vi "Teleop.vi"(10 "Match Info":T1={"Autonomous Elapsed Seconds"=0.0, "TeleOp Elapsed Seconds"=0.0, "Disabled Elapsed Seconds"=0.0, "Visited Autonomous"=FALSE, "Visited TeleOp"=FALSE, "Visited Disabled"=FALSE, "Autonomous Settings"={"Autonomous Style"=enum."Independent", "VI Refnum"=refnum}}, 11 "Call Context":T2) -> ()   [LabVIEW 2014]
doc: "This VI is called for each TeleOp packet received from the DS where the robot is not disabled. It is often used to read from the joysticks and update I/O or to update setpoints for timed control loops. It should complete and return within 20 milliseconds or it may miss DS packets."
uses:
  <vilib>/Rock Robotics/WPI/DriverStation/WPI_DriverStationDerivedRobotMode.ctl
  <vilib>/Rock Robotics/WPI/DriverStation/WPI_DriverStationMatch Info.ctl
  <vilib>/Rock Robotics/WPI/Joystick/WPI_JoystickGetSetRefNum.vi
  <vilib>/Rock Robotics/Network Tables/SD Write Boolean Array.vi
  <vilib>/Rock Robotics/Network Tables/SD Write Numeric Array.vi
panel:
  out "Right Motor":dbl(graph)
  out "Left Motor":dbl(graph)
  out "Left Sensor Velocity":dbl
  out "Right Sensor Velocity":dbl
  out "Waveform Chart":dbl(graph)
  in  "SET VALUE":dbl
  in  "TRUE - JOY\nFALSE - SET VALUE":bool
  out "X Value":dbl
  out "Y value":dbl
  out "Right Sensor Velocity In inches per second 2":dbl(graph)
  out "Left Sensor Velocity In inches per second":dbl(graph)
  out "Applied Throttle":dbl(graph)
  out "Motor Output":dbl
  # "Sensor Velocity is in ticks per 100ms"
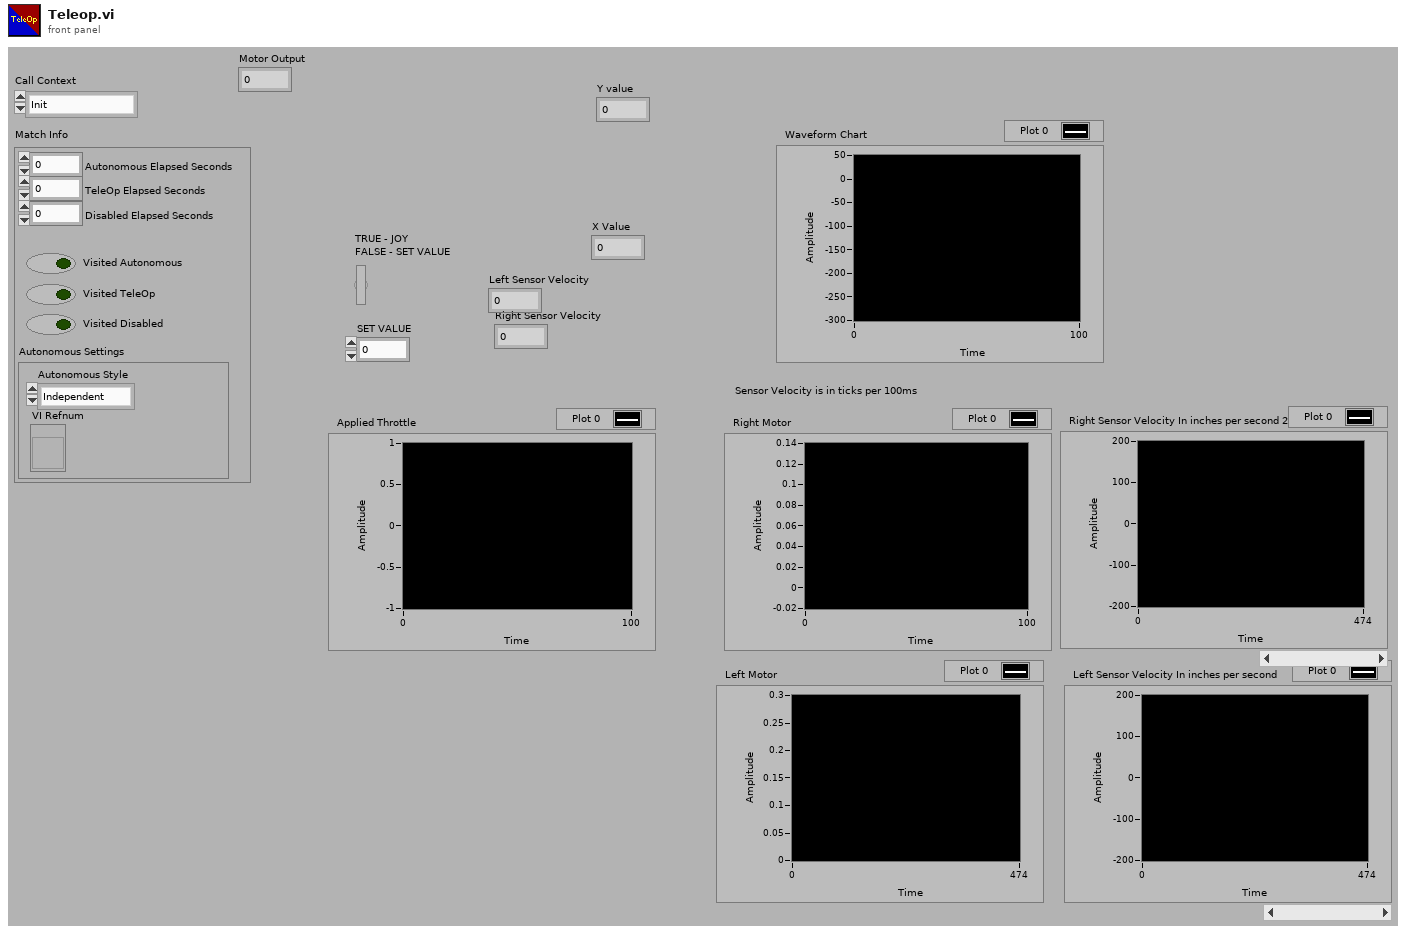
[diagram p1: front panel]
types:
  T1 = typedef "WPI_DriverStationMatch Info.ctl" = cluster{"Autonomous Elapsed Seconds":dbl, "TeleOp Elapsed Seconds":dbl, "Disabled Elapsed Seconds":dbl, "Visited Autonomous":bool, "Visited TeleOp":bool, "Visited Disabled":bool, "Autonomous Settings":cluster{"Autonomous Style":enum16{"Iterative", "Independent"}, "VI Refnum":refnum<vi>}}
  T2 = typedef "WPI_DriverStationDerivedRobotMode.ctl" = enum16{"Init", "Execute", "Stop"}
  T3 = typedef "WPI_MotorControlDeviceRef.ctl" = cluster{"DeviceStatus":errorcluster, "Type":T4, "PWM":cluster{"Controller":T5, "PWM Channel":T6, "DeadBand":T7}, "CAN":cluster{"Device Number":u8, "Control Mode":T8, "Semaphore":T9, "Max Vout":dbl, "TalonSRX Control Mode":T10}, "Invert":bool, "TransformRef":T11, "InvTransformRef":T11}
  T4 = typedef "WPI_MotorControlType.ctl" = enum16{"PWM", "CAN", "CANTalonSRX"}
  T5 = typedef "FPGA_TypedefDigitalModule.ctl" = enum16{"Controller 1"}
  T6 = typedef "FPGA_DIOPWMChannel.ctl" = enum8{"PWM 0", "PWM 1", "PWM 2", "PWM 3", "PWM 4", "PWM 5", "PWM 6", "PWM 7", "PWM 8", "PWM 9", "PWM MXP 0", "PWM MXP 1", "PWM MXP 2", "PWM MXP 3", "PWM MXP 4", "PWM MXP 5", "PWM MXP 6", "PWM MXP 7", "PWM MXP 8", "PWM MXP 9", "Invalid"}
  T7 = typedef "WPI_PWMDeadband.ctl" = cluster{"Name":string, "maxPositivePwm":i32, "minPositivePwm":i32, "centerPwm":i32, "maxNegativePwm":i32, "minNegativePwm":i32, "angularRange":u16}
  T8 = typedef "WPI_CANJaguar_ControlMode.ctl" = enum8{"Percent VBus", "Current", "Speed", "Position", "Voltage"}
  T9 = typedef "Semaphore RefNum" = refnum<k1>
  T10 = typedef "WPI_CANTalonSRX_APIControlMode.ctl" = enum8{"Percent VBus", "Speed", "Position", "Slave", "Unchanged / Invalid"}
  T11 = typedef "WPI_PWMTransform_ConPane.ctl" = refnum<vi>
  T12 = typedef "WPI_JoystickDevRef.ctl" = cluster{"Device":T13}
  T13 = typedef "WPI_JoystickDeviceEnum.ctl" = enum16{"USB 0", "USB 1", "USB 2", "USB 3", "USB 4", "USB 5"}
  T14 = typedef "WPI_CANTalonSRX_GlobalStatus.ctl" = cluster{"Applied Throttle":dbl, "Module Enabled":bool, "CAN Error":errorcluster, "Closed Loop Error":dbl, "Forward Limit Switch Closed":bool, "Reverse Limit Switch Closed":bool, "Sensor Position":dbl, "Sensor Velocity":dbl, "Current":dbl, "Sticky Fault - Over Temp":bool, "Sticky Fault - Under Voltage":bool, "Sticky Fault - Forward Limit":bool, "Sticky Fault - Reverse Limit":bool, "Sticky Fault - Forward Soft Limit":bool, "Sticky Fault - Reverse Soft Limit":bool, "Brake is Enabled":bool, "Encoder Position":dbl, "Encoder Velocity":dbl, "Encoder Index Count":dbl, "Encoder A Pin State":bool, "Encoder B Pin State":bool, "Encoder Index Pin State":bool, "Analog In":dbl, "Analog In Velocity":dbl, "Temperature (C)":dbl, "Battery Voltage":dbl}
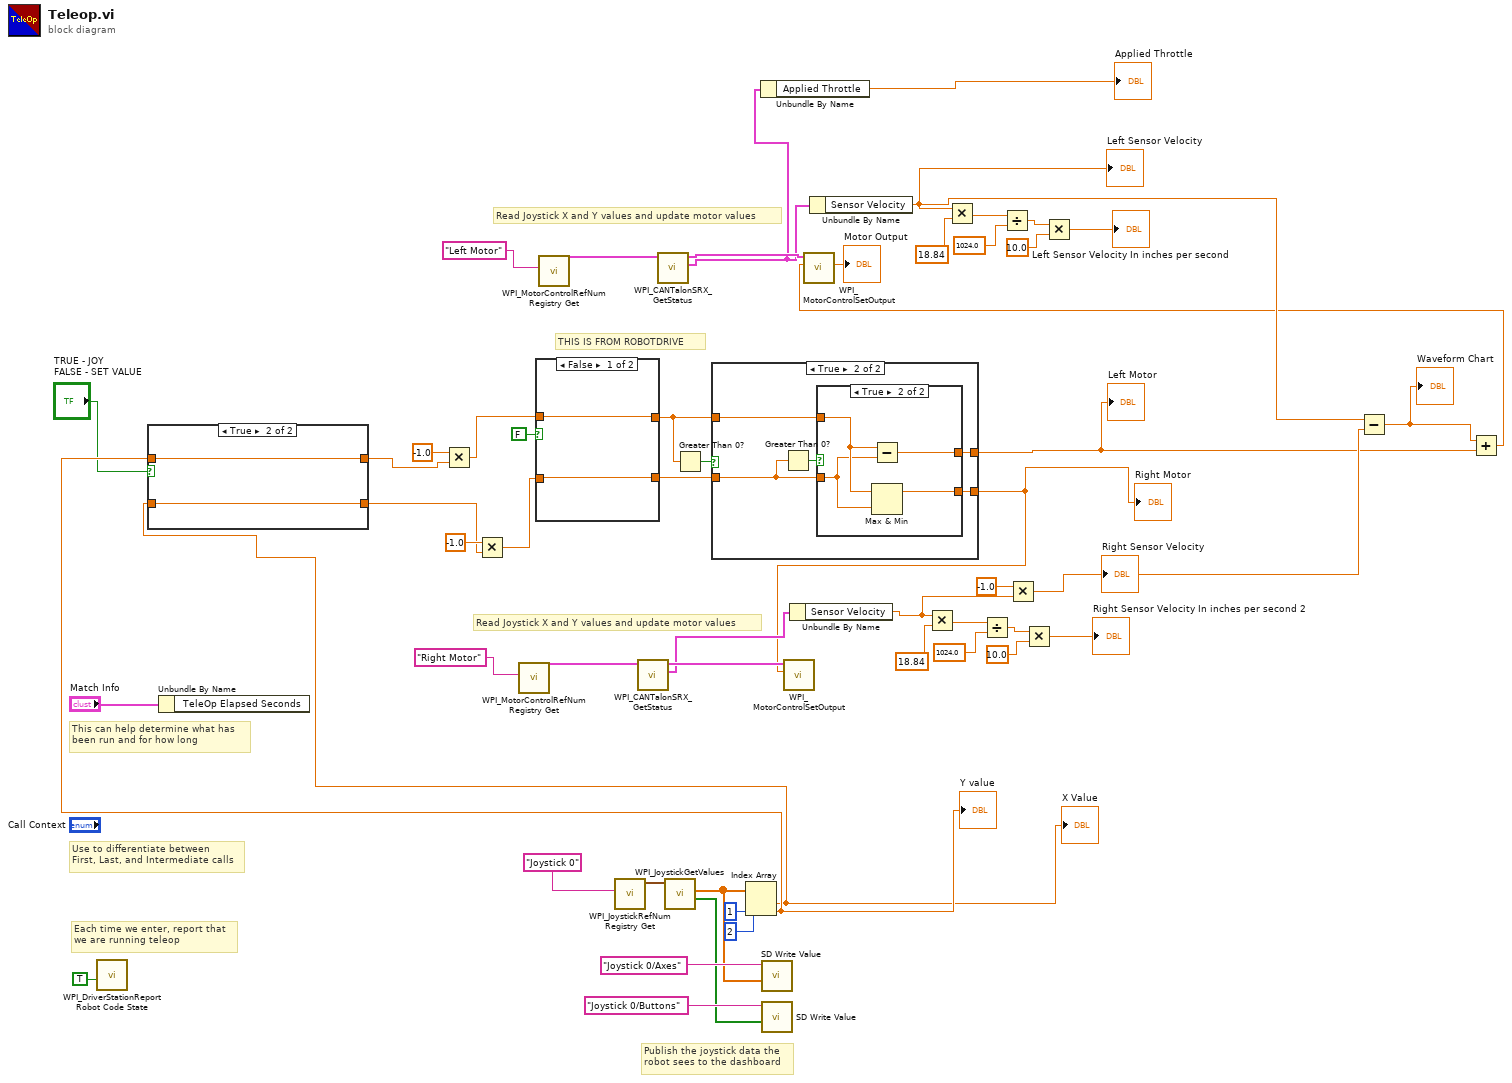
[diagram p0: block diagram]
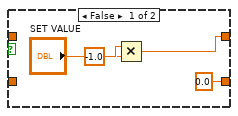
[diagram p2: hidden frame]
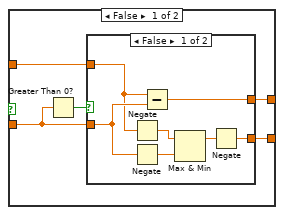
[diagram p3: hidden frame]
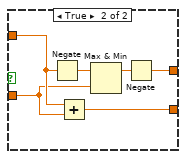
[diagram p4: hidden frame]
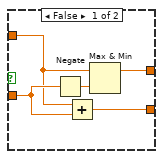
[diagram p5: hidden frame]
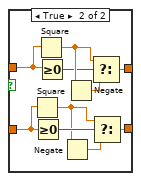
[diagram p6: hidden frame]
diagram:
  # "THIS IS FROM ROBOTDRIVE"
  # "Read Joystick X and Y values and update motor values"
  # "Publish the joystick data the\nrobot sees to the dashboard"
  # "Each time we enter, report that\nwe are running teleop"
  # "Use to differentiate between\nFirst, Last, and Intermediate calls"
  # "This can help determine what has\nbeen run and for how long"
  # "Read Joystick X and Y values and update motor values"
  n1 = call <vilib>:"WPI_DriverStationReport Robot Code State.vi"("TeleOp"=TRUE ("Autonomous")) -> ()  [unwired: 10 in, 1 out]
  n2 = Unbundle By Name("Match Info") -> ()  [unwired: 1 out]
  n3 = call <vilib>:"WPI_MotorControlRefNum Registry Get.vi"("refnum name"="Right Motor") -> ("MotorControlDevRef"=w32:T3)  [unwired: 9 in, 1 out]
  n4 = call <vilib>:"WPI_MotorControlRefNum Registry Get.vi"("refnum name"="Left Motor") -> ("MotorControlDevRef"=w43:T3)  [unwired: 9 in, 1 out]
  n5 = call <vilib>:"WPI_JoystickRefNum Registry Get.vi"("refnum name"="Joystick 0") -> ("JoystickDevRef"=w51:T12)  [unwired: 1 in, 9 out]
  n6 = call <vilib>:"WPI_CANTalonSRX_GetStatus.vi"("CAN Talon SRX Ref"=w32) -> ("Talon SRX Status"=w30:T14, "CAN Talon SRX Ref Out"=w31:T3)  [unwired: 8 in, 1 out]
  n7 = call <vilib>:"WPI_CANTalonSRX_GetStatus.vi"("CAN Talon SRX Ref"=w43) -> ("Talon SRX Status"=w40:T14, "CAN Talon SRX Ref Out"=w42:T3)  [unwired: 8 in, 1 out]
  n8 = call <vilib>:"WPI_JoystickGetValues.vi"("JoystickDevRef"=w51) -> ("Buttons"=w46:bool[], "Axes"=w48:dbl[])  [unwired: 6 in, 3 out]
  n9 = Index Array(array=w48, index #1=2 ("index"), index #2=1 ("index")) -> (element #1=w11:dbl, element #2=w13:dbl)
  "Y value" <- w13
  "X Value" <- w11
  n10 = case shown="True" "TRUE - JOY\nFALSE - SET VALUE" {
    tunnel: w13 -> [_ w59]
    tunnel: [w56 w59] -> w12
    tunnel: w11 -> [_ w58]
    tunnel: [0.0 ("upper limit") w58] -> w10
    frame False {
      n11 = Multiply(x="SET VALUE", y=-1.0) -> (x*y=w56:dbl)
    }
    frame True {
    }
  }
  n12 = Multiply(x=-1.0, y=w12) -> (x*y=w17:dbl)
  n13 = Multiply(x=-1.0, y=w10) -> (x*y=w19:dbl)
  n14 = case shown="False" FALSE {
    tunnel: [w60 w71] -> w21
    tunnel: [w61 w70] -> w22
    tunnel: w19 -> [w60 w69]
    tunnel: w17 -> [w61 w68]
    frame False {
    }
    frame True {
      n15 = Square(x=w69) -> (x^2=w66:dbl)
      n16 = Greater Or Equal To 0?(x=w69) -> (x >= 0?=w67:bool)
      n17 = Square(x=w68) -> (x^2=w63:dbl)
      n18 = Greater Or Equal To 0?(x=w68) -> (x >= 0?=w62:bool)
      n19 = Negate(x=w66) -> (-x=w65:dbl)
      n20 = Negate(x=w63) -> (-x=w64:dbl)
      n21 = Select(t=w63, s=w62, f=w64) -> (s? t:f=w70:dbl)
      n22 = Select(t=w66, s=w67, f=w65) -> (s? t:f=w71:dbl)
    }
  }
  n23 = Greater Than 0?(x=w22) -> (x > 0?=w23:bool)
  n24 = case shown="True" w23 {
    tunnel: w21 -> [w75 w93]
    tunnel: w22 -> [w74 w92]
    tunnel: [w73 w91] -> w2
    tunnel: [w72 w90] -> w1
    frame False {
      n25 = Greater Than 0?(x=w75) -> (x > 0?=w76:bool)
      n26 = case shown="False" w76 {
        tunnel: w75 -> [w83 w85]
        tunnel: w74 -> [w81 w86]
        tunnel: [w77 w87] -> w73
        tunnel: [w78 w84] -> w72
        frame False {
          n27 = Negate(x=w81) -> (-x=w82:dbl)
          n28 = Negate(x=w83) -> (-x=w80:dbl)
          n29 = Subtract(x=w81, y=w83) -> (x-y=w77:dbl)
          n30 = Max & Min(x=w82, y=w80) -> (max(x,y)=w79:dbl)  [unwired: 1 out]
          n31 = Negate(x=w79) -> (-x=w78:dbl)
        }
        frame True {
          n32 = Negate(x=w86) -> (-x=w89:dbl)
          n33 = Add(x=w86, y=w85) -> (x+y=w84:dbl)
          n34 = Max & Min(x=w89, y=w85) -> (max(x,y)=w88:dbl)  [unwired: 1 out]
          n35 = Negate(x=w88) -> (-x=w87:dbl)
        }
      }
    }
    frame True {
      n36 = Greater Than 0?(x=w93) -> (x > 0?=w94:bool)
      n37 = case shown="True" w94 {
        tunnel: w93 -> [w99 w101]
        tunnel: w92 -> [w96 w102]
        tunnel: [w97 w100] -> w91
        tunnel: [w95 w103] -> w90
        frame False {
          n38 = Negate(x=w99) -> (-x=w98:dbl)
          n39 = Add(x=w96, y=w99) -> (x+y=w95:dbl)
          n40 = Max & Min(x=w96, y=w98) -> (max(x,y)=w97:dbl)  [unwired: 1 out]
        }
        frame True {
          n41 = Subtract(x=w102, y=w101) -> (x-y=w100:dbl)
          n42 = Max & Min(x=w102, y=w101) -> (max(x,y)=w103:dbl)  [unwired: 1 out]
        }
      }
    }
  }
  "Left Motor" <- w2
  "Right Motor" <- w1
  n43 = Unbundle By Name(w40) -> ("Applied Throttle"=→"Applied Throttle":dbl)
  n44 = call-poly <vilib>:"SD Write Value.vi"("Numeric Array"=w48, "Name"="Joystick 0/Axes") -> ()  [unwired: 8 in, 2 out]
  n45 = call-poly <vilib>:"SD Write Value.vi"("Boolean Array"=w46, "Name"="Joystick 0/Buttons") -> ()  [unwired: 8 in, 2 out]
  n46 = call <vilib>:"WPI_MotorControlSetOutput.vi"("Output"=w1, "MotorControlDevRef"=w31) -> ()  [unwired: 7 in, 3 out]
  n47 = Unbundle By Name(w30) -> ("Sensor Velocity"=w5:dbl)
  n48 = Unbundle By Name(w40) -> ("Sensor Velocity"=w8:dbl)
  "Left Sensor Velocity" <- w8
  n49 = Multiply(x=w5, y=18.84) -> (x*y=w28:dbl)
  n50 = Multiply(x=w8, y=18.84) -> (x*y=w38:dbl)
  n51 = Divide(x=w28, y=1024.0) -> (x/y=w26:dbl)
  n52 = Divide(x=w38, y=1024.0) -> (x/y=w36:dbl)
  n53 = Multiply(x=-1.0, y=w5) -> (x*y=w3:dbl)
  "Right Sensor Velocity" <- w3
  n54 = Multiply(x=w26, y=10.0) -> (x*y=→"Right Sensor Velocity In inches per second 2":dbl)
  n55 = Multiply(x=w36, y=10.0) -> (x*y=→"Left Sensor Velocity In inches per second":dbl)
  n56 = Subtract(x=w8, y=w3) -> (x-y=w6:dbl)
  "Waveform Chart" <- w6
  n57 = Add(x=w6, y=w2) -> (x+y=w7:dbl)
  n58 = call <vilib>:"WPI_MotorControlSetOutput.vi"("Output"=w7, "MotorControlDevRef"=w42) -> ("Motor Output"=→"Motor Output":dbl)  [unwired: 7 in, 2 out]
